vi "init.vi"(8 "error in (no error)":errorcluster, 11 "DistanceGaugeTC in":refnum<class "DistanceGaugeTC.lvclass">) -> (0 "error out":errorcluster, 3 "DistanceGaugeTC out":refnum<class "DistanceGaugeTC.lvclass">)   [LabVIEW 2013, in "DistanceGaugeTC.lvclass"]
uses:
  DistanceGaugeTC.lvclass
  <userlib>/Common/Devices/DistanceGauge/Config/Distance Gauge.ctl
  <userlib>/Common/SerialProtocols/Configuration/SerialConfig.ctl
  <userlib>/Common/SerialProtocols/Configuration/SerialProtocol.ctl
  <userlib>/Common/SerialProtocols/Configuration/ProtocolParameters.ctl
  <userlib>/Common/SerialProtocols/Configuration/SerialMessageParameters.ctl
  <userlib>/Common/Devices/DistanceGauge/Config/ChannelsToRead.ctl
  <userlib>/Common/Devices/DistanceGauge/DistanceGauge/DistanceGauge.lvclass/DistanceGauge.ctl
  <userlib>/Common/Devices/DistanceGauge/DistanceGauge/DistanceGauge.lvclass
  <userlib>/Common/Devices/DistanceGauge/DistanceGauge.lvlib
  <userlib>/Common/SerialProtocols/SerialProtocols.lvlib
  ConfigurationThisComponent/ConfigurationThisComponent.lvclass
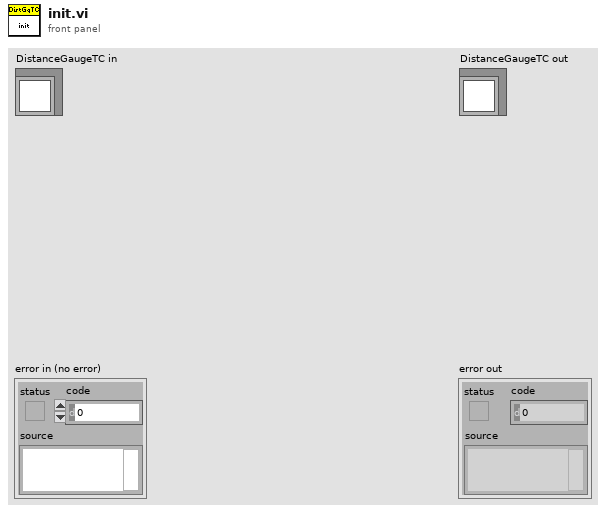
[diagram p1: front panel]
types:
  T1 = typedef "DistanceGauge.lvlib/Distance Gauge.ctl" = cluster{"Serial":T2, "Channels To Read":T6}
  T2 = typedef "SerialProtocols.lvlib/SerialConfig.ctl" = cluster{"Serial Protocol":T3, "Protocol Parameters":T4, "Serial Message Parameters":T5}
  T3 = typedef "SerialProtocols.lvlib/SerialProtocol.ctl" = enum16{"RS232", "RS485", "SerialSimulator"}
  T4 = typedef "SerialProtocols.lvlib/ProtocolParameters.ctl" = cluster{"VISA resource name":refnum<visa-resource-name>, "Baud Rate":u32, "Data Bits":u16, "Parity":enum16{"None", "Odd", "Even", "Mark", "Space"}, "Flow Control":u16, "Stop Bits":u16, "Timeout (ms)":u32}
  T5 = typedef "SerialProtocols.lvlib/SerialMessageParameters.ctl" = cluster{"Byte Count":u32, "Enable Termination Character":bool, "Termination Char":u8}
  T6 = typedef "DistanceGauge.lvlib/ChannelsToRead.ctl" = i32[]
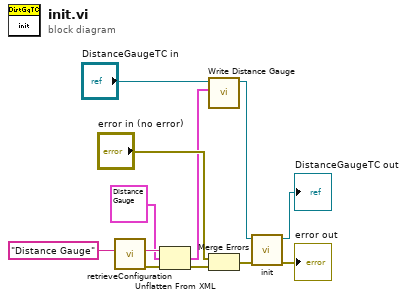
[diagram p0: block diagram]
diagram:
  n1 = call "retrieveConfiguration.vi"("configName"="Distance Gauge") -> ("error out"=w7:errorcluster, "xmlConfig"=w8:string)  [unwired: 8 in, 1 out]
  n2 = Unflatten From XML(xml string=w8, type=T1 {"Serial"={"Serial Protocol"=enum."RS232", "Protocol Parameters"={"VISA resource name"="", "Baud Rate"=0, "Data Bits"=0, "Parity"=enum."None", "Flow Control"=0, "Stop Bits"=0, "Timeout (ms)"=0}, "Serial Message Parameters"={"Byte Count"=0, "Enable Termination Character"=FALSE, "Termination Char"=0}}, "Channels To Read"=[]} ("Distance Gauge"), error in (no error)=w7) -> (value=w1:T1, error out=w10:errorcluster)
  n3 = call <userlib>:"Write Distance Gauge.vi"("Distance Gauge"=w1, "DistanceGauge in"="DistanceGaugeTC in") -> ("DistanceGauge out"=w4:refnum<class "DistanceGaugeTC.lvclass">)  [unwired: 9 in]
  n4 = Merge Errors("error in (no error)", w10) -> (w2:errorcluster)
  n5 = call-parent "init.vi"("error in (no error)"=w2, "DistanceGauge in"=w4) -> ("error out"=→"error out":errorcluster, "DistanceGauge out"=→"DistanceGaugeTC out":refnum<class "DistanceGaugeTC.lvclass">)  [unwired: 8 in]
